vi "DataRead.vi"(7 "base path":path=path "C:/Data/Pega/Referans", 9 "Tekrar":i32, 10 "Excel_In":dbl[][](array[numeric]), 11 "Adet":i32) -> ()   [LabVIEW 2021]
uses:
  <vilib>/Utility/file.llb/Write Delimited Spreadsheet (string).vi
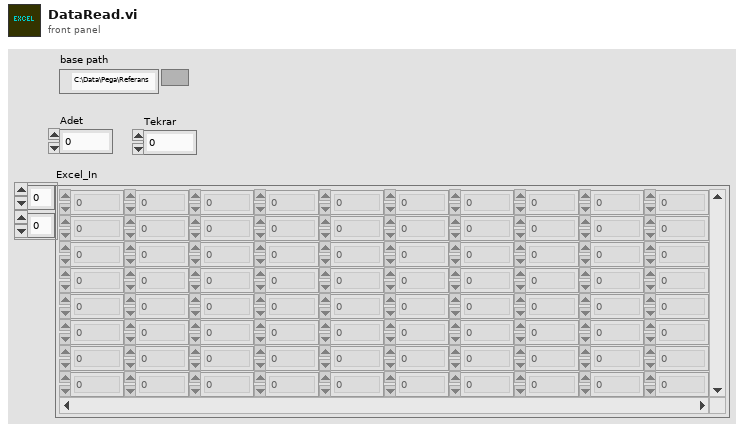
[diagram p1: front panel]
types:
  T1 = enum16{"open", "replace", "create", "open or create", "replace or create", "replace or create with confirmation"}
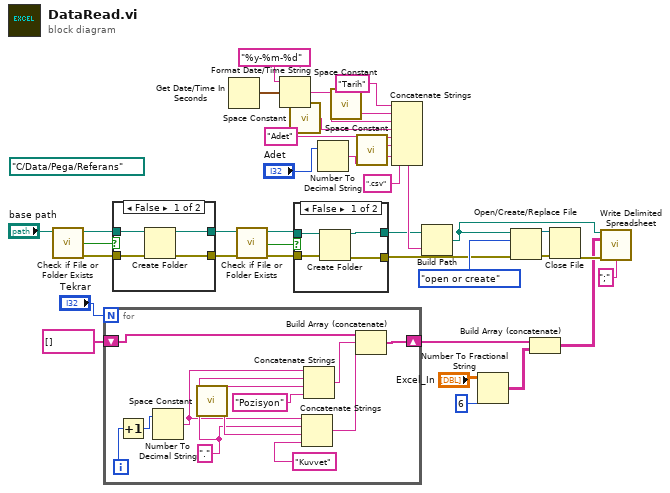
[diagram p0: block diagram]
diagram:
  (unwired) path "C:/Data/Pega/Referans" ("base path")
  n1 = call <vilib>:"Check if File or Folder Exists.vi"("path"="base path") -> ("error out"=w32:errorcluster, "file or folder exists?"=w34:bool, "dup path"=w33:path)  [unwired: 8 in]
  n2 = for {
    N: "Tekrar" -> [_]
    shift-right: [w47] -> w11
    shift-left: string[] [] -> [w46]
    i -> [w42]
    w38 = "."
    n3 = Increment(x=w42) -> (x+1=w43:i32)
    n4 = Number To Decimal String(number=w43) -> (decimal integer string=w37:string)  [unwired: 1 in]
    n5 = call <vilib>:"Space Constant.vi"() -> ("String"=w40:string)
    n6 = Concatenate Strings(w37, w38, w40, "Kuvvet") -> (w44:string)
    n7 = Concatenate Strings(w37, w38, w40, "Pozisyon") -> (w45:string)
    n8 = Build Array (concatenate)(w46, w45, w44) -> (w47:string[])
  }
  n9 = case shown="False" w34 {
    tunnel: w33 -> [w51 w53]
    tunnel: [w50 w53] -> w6
    tunnel: w32 -> [w49 w52]
    tunnel: [w48 w52] -> w28
    frame False {
      n10 = Create Folder(path (use dialog)=w51, error in=w49) -> (created path=w50:path, error out=w48:errorcluster)  [unwired: 1 in, 1 out]
    }
    frame True {
    }
  }
  n11 = Get Date/Time In Seconds() -> (seconds since 1Jan1904=w36:timestamp)
  n12 = call <vilib>:"Check if File or Folder Exists.vi"("error in (no error)"=w28, "path"=w6) -> ("error out"=w29:errorcluster, "file or folder exists?"=w31:bool, "dup path"=w30:path)  [unwired: 7 in]
  n13 = Format Date/Time String(time format string (%c)="%y-%m-%d", seconds (now)=w36) -> (date/time string=w4:string)  [unwired: 1 in]
  n14 = call <vilib>:"Space Constant.vi"() -> ("String"=w5:string)
  n15 = case shown="False" w31 {
    tunnel: w30 -> [w57 w59]
    tunnel: [w56 w59] -> w25
    tunnel: w29 -> [w55 w58]
    tunnel: [w54 w58] -> w22
    frame False {
      n16 = Create Folder(path (use dialog)=w57, error in=w55) -> (created path=w56:path, error out=w54:errorcluster)  [unwired: 1 in, 1 out]
    }
    frame True {
    }
  }
  n17 = Number To Decimal String(number="Adet") -> (decimal integer string=w16:string)  [unwired: 1 in]
  n18 = call <vilib>:"Space Constant.vi"() -> ("String"=w3:string)
  n19 = call <vilib>:"Space Constant.vi"() -> ("String"=w26:string)
  n20 = Concatenate Strings("Tarih" ("string"), w3, w4, w5, "Adet" ("string"), w26, w16, ".csv" ("string")) -> (w27:string)
  n21 = Build Path(base path=w25, name or relative path=w27) -> (appended path=w19:path)
  n22 = Number To Fractional String(number="Excel_In", precision (6)=i16 6) -> (F-format string=w8:string[][])  [unwired: 2 in]
  n23 = Open/Create/Replace File(file path (use dialog)=w19, error in=w22, operation (0:open)=T1."open or create") -> (refnum out=w21:refnum<file>, error out=w20:errorcluster)  [unwired: 3 in, 1 out]
  n24 = Build Array (concatenate)(w11, w8) -> (w10:string[][])
  n25 = Close File(refnum=w21, error in=w20) -> (error out=w18:errorcluster)  [unwired: 1 out]
  n26 = call-poly <vilib>:"Write Delimited Spreadsheet.vi"("file path (dialog if empty)"=w19, "2D data"=w10, "error in (no error)"=w18, "delimiter (\\t)"=";" ("delimiter (\\t)")) -> ()  [unwired: 10 in, 2 out]
